vi "WfmMain.vi"() -> ()   [LabVIEW 2012]
doc: "Use this template to build a simple state machine design pattern. Each state executes code and determines which state to transition to."
uses:
  controls/WfmState.ctl
  controls/WfmData.ctl
panel:
  out "Waveform Graph":dbl[](graph)
  in  "Log to File":bool
  in  "Acquire Waveform":bool
  in  "Stop Button":bool
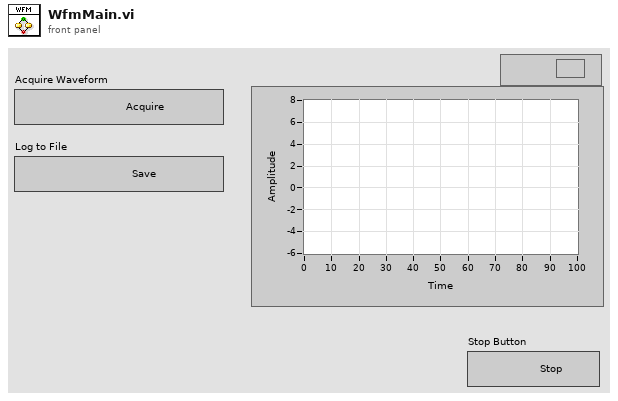
[diagram p1: front panel]
types:
  T1 = typedef "WfmData.ctl" = cluster{"Array":dbl[]}
  T2 = typedef "WfmState.ctl" = enum16{"Initialize", "Wait for Event", "Acquire Waveform", "Log to File", "Stop"}
  T3 = enum16{"uniform white", "uniform+uniform", "Gaussian white", "sine", "square"}
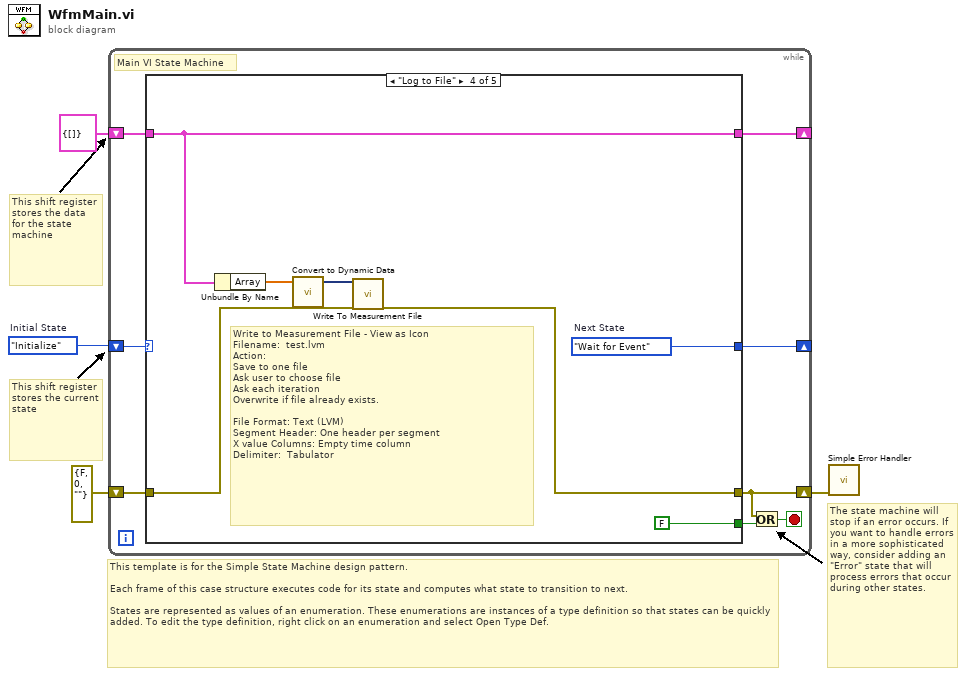
[diagram p0: block diagram]
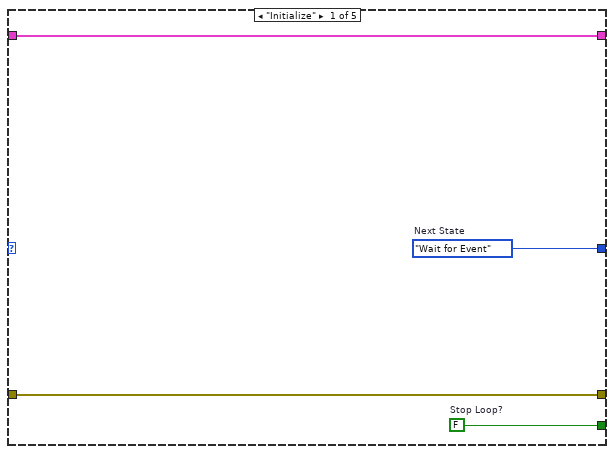
[diagram p2: hidden frame]
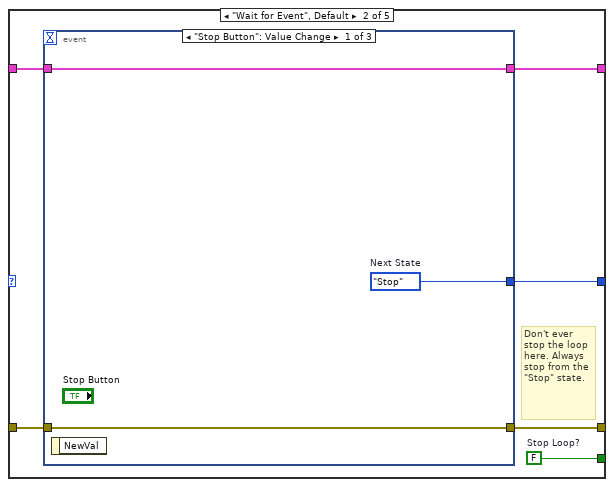
[diagram p3: hidden frame]
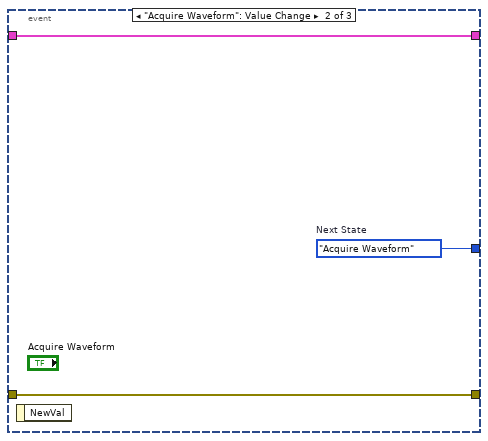
[diagram p4: hidden frame]
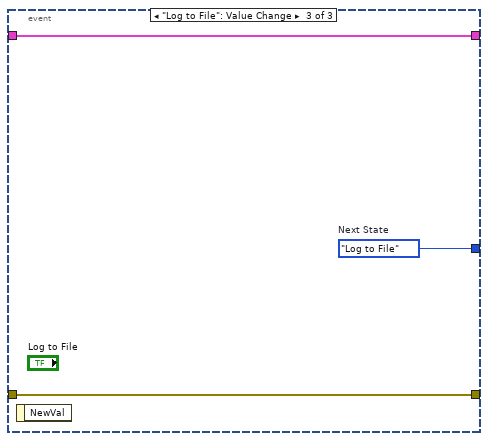
[diagram p5: hidden frame]
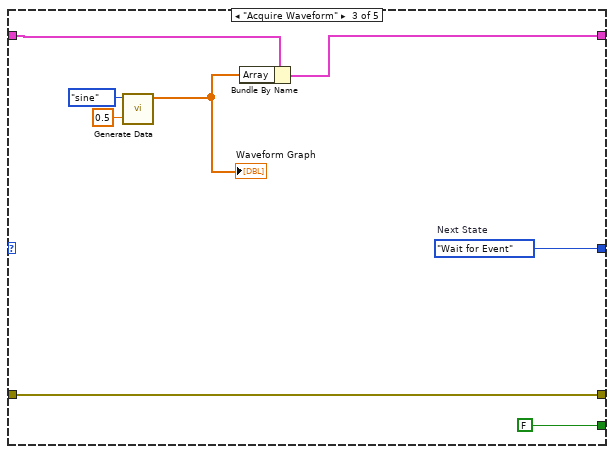
[diagram p6: hidden frame]
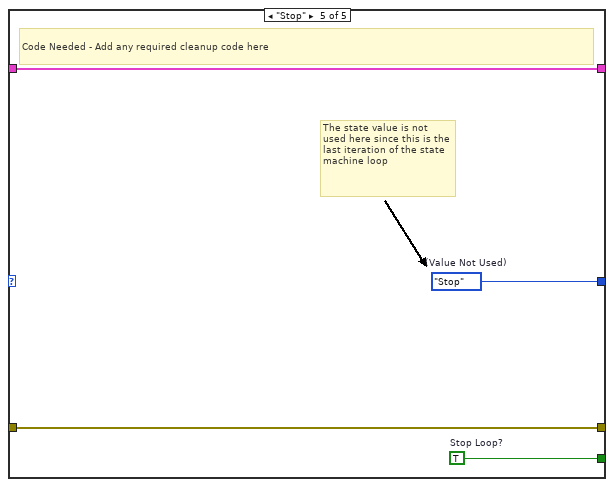
[diagram p7: hidden frame]
diagram:
  w4 = WfmState."Initialize"  # Initial State
  # "The state machine will stop if an error occurs. If you want to handle errors in a more sophisticated way, consider adding an \"Error\" state that will process errors that occur during other states."
  # "This shift register\nstores the data for the state machine"
  # "This template is for the Simple State Machine design pattern.\n\nEach frame of this case structure executes code for its state and computes what state to transition to next.\n\nStates are represented as values of an enumeration. These enumerations are instances of a type definition so that states can be quickly added. To edit the type definition, right click on an enumeration and select Open Type Def."
  # "This shift register\nstores the current\nstate"
  n1 = while {
    shift-right: [w11] -> _
    shift-left: w4 -> [w12]
    shift-right: [w9] -> _
    shift-left: T1 {"Array"=[]} ("Data") -> [w10]
    shift-right: [w5] -> w1
    shift-left: errorcluster {"status"=FALSE, "code"=0, "source"=""} ("error constant") -> [w8]
    stop <- w6 stop-if-true
    # "Main VI State Machine"
    n2 = case shown="\"Log to File\"" w12 {
      tunnel: [w16 w22 w39 w46 w50] -> w11
      tunnel: [w15 w21 FALSE ("Stop Loop?") FALSE ("Stop Loop?") w48] -> w7
      tunnel: w10 -> [w13 w20 w37 w44 w49]
      tunnel: [w13 w19 w36 w44 w49] -> w9
      tunnel: w8 -> [w14 w18 w34 w41 w47]
      tunnel: [w14 w17 w34 w40 w47] -> w5
      frame "Initialize" {
        w15 = FALSE  # Stop Loop?
        w16 = WfmState."Wait for Event"  # Next State
      }
      frame "Wait for Event", Default {
        w21 = FALSE  # Stop Loop?
        # "Don't ever stop the loop here. Always stop from the \"Stop\" state."
        n3 = event shown="[0] \"Stop Button\": Value Change" {
          selector: _ -> [_ _ _]
          dyn-events: _ -> [_ _ _]
          timeout: _ -> [_ _ _]
          tunnel: [w25 w28 w31] -> w22
          tunnel: w20 -> [w24 w26 w29]
          tunnel: [w24 w26 w29] -> w19
          tunnel: w18 -> [w23 w27 w30]
          tunnel: [w23 w27 w30] -> w17
          event "Stop Button": Value Change {
            w25 = WfmState."Stop"  # Next State
            n4 = event-data() -> ()  [unwired: 1 in, 1 out]
          }
          event "Acquire Waveform": Value Change {
            w28 = WfmState."Acquire Waveform"  # Next State
            n5 = event-data() -> ()  [unwired: 1 in, 1 out]
          }
          event "Log to File": Value Change {
            w31 = WfmState."Log to File"  # Next State
            n6 = event-data() -> ()  [unwired: 1 in, 1 out]
          }
        }
      }
      frame "Acquire Waveform" {
        w39 = WfmState."Wait for Event"  # Next State
        n7 = call "Generate Data.vi"("noise (rms)"=0.5, "signal"=T3."sine") -> ("Y"=w35:dbl[])  [unwired: 8 in, 1 out]
        "Waveform Graph" <- w35
        n8 = Bundle By Name(cluster=w37, "Array"=w35) -> (w36:T1)
      }
      frame "Log to File" {
        w46 = WfmState."Wait for Event"  # Next State
        # "Write to Measurement File - View as Icon\nFilename:  test.lvm\nAction:\nSave to one file\nAsk user to choose file\nAsk each iteration\nOverwrite if file already exists.\n\nFile Format: Text (LVM)\nSegment Header: One header per segment\nX value Columns: Empty time column\nDelimiter:  Tabulator"
        n9 = Unbundle By Name(w44) -> ("Array"=w43:dbl[])
        n10 = call "Convert to Dynamic Data"("Array"=w43) -> ("Dynamic Data Type"=w42:dynamicdata)  [unwired: 3 in]
        n11 = call "Write To Measurement File"("Signals"=w42, "error in (no error)"=w41) -> ("error out"=w40:errorcluster)  [unwired: 15 in, 2 out]
      }
      frame "Stop" {
        w48 = TRUE  # Stop Loop?
        w50 = WfmState."Stop"  # (Value Not Used)
        # "Code Needed - Add any required cleanup code here"
        # "The state value is not used here since this is the last iteration of the state machine loop"
      }
    }
    n12 = Or(x=w5, y=w7) -> (x .or. y?=w6:bool)
  }
  n13 = call <vilib>:"Simple Error Handler.vi"("error in (no error)"=w1) -> ()  [unwired: 4 in, 5 out]
